vi "[RT] Send eHS CPU Constants.vi"(8 "Error In":errorcluster, 9 "eHS SW Constants":bool[](array[boolean]), 10 "eHS Constant Inputs":sgl[](array[numeric]), 11 "FPGA Reference In":T1) -> (0 "Error Out":errorcluster, 3 "FPGA Reference Out":T1)   [LabVIEW 2017]
uses:
  Controls/eHS FPGA Ref.ctl
  <vilib>/Utility/error.llb/Error Cluster From Error Code.vi
  <vilib>/rvi/errors/niLvFpgaAdjustHostInterfaceError.vi
  <vilib>/rvi/interface/nirviReadWriteControl/nirviReadWriteControl.xnode
  NiFpgaLv.dll
  <vilib>/rvi/interface/Simulation/niFpgaSimulationCallBeginRW.vi
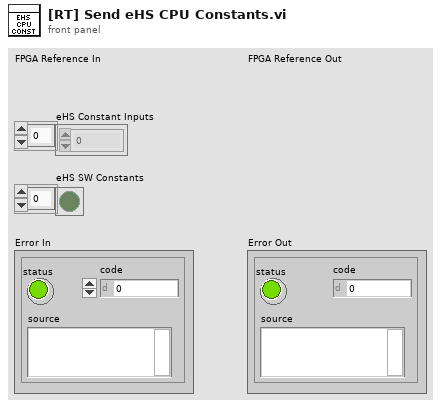
[diagram p1: front panel]
types:
  T1 = typedef "eHS FPGA Ref.ctl" = refnum<k20>
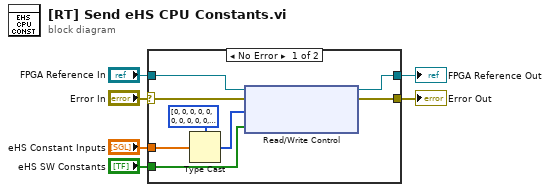
[diagram p0: block diagram]
diagram:
  n1 = case shown="No Error" "Error In" {
    selector: "Error In" -> [w7 w15]
    tunnel: [w14 w16] -> w6
    tunnel: [w13 w15] -> w5
    tunnel: "eHS Constant Inputs" -> [w12 _]
    tunnel: "FPGA Reference In" -> [w10 w16]
    tunnel: "eHS SW Constants" -> [w8 _]
    frame No Error {
      n2 = Type Cast(type=u32[] [0, 0, 0, 0, 0, 0, 0, 0, 0, 0, 0, 0, 0, 0, 0, 0, 0, 0, 0, 0, 0, 0, 0, 0, 0, 0, 0, 0, 0, 0, 0, 0], x=w12) -> (*(type *) &x=w9:u32[])
      n3 = xnode "Read/Write Control"("FPGA VI Reference In"=w10, "error in"=w7, "eHS Input (CPU)"=w9, "eHS Switches (CPU)"=w8) -> ("FPGA VI Reference Out"=w14:T1, "error out"=w13:errorcluster)
    }
    frame Error {
    }
  }
  "FPGA Reference Out" <- w6
  "Error Out" <- w5
